vi "Initialize.vi"(8 "error in":errorcluster, 10 "Btr0Btr1":u16=28 format="%.0x", 11 "Channel":u16=65 format="%x") -> (0 "error out":errorcluster, 3 "Channel out":u16=81, 5 "function return":u32)   [LabVIEW 2023, in "PCAN API.lvlib"]
doc: "This VI is used for initializing a CAN port."
uses:
  PCAN API.lvlib
  PCAN2023/PCAN2023.lvlib
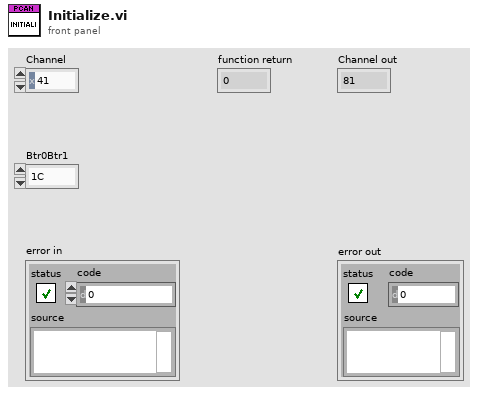
[diagram p1: front panel]
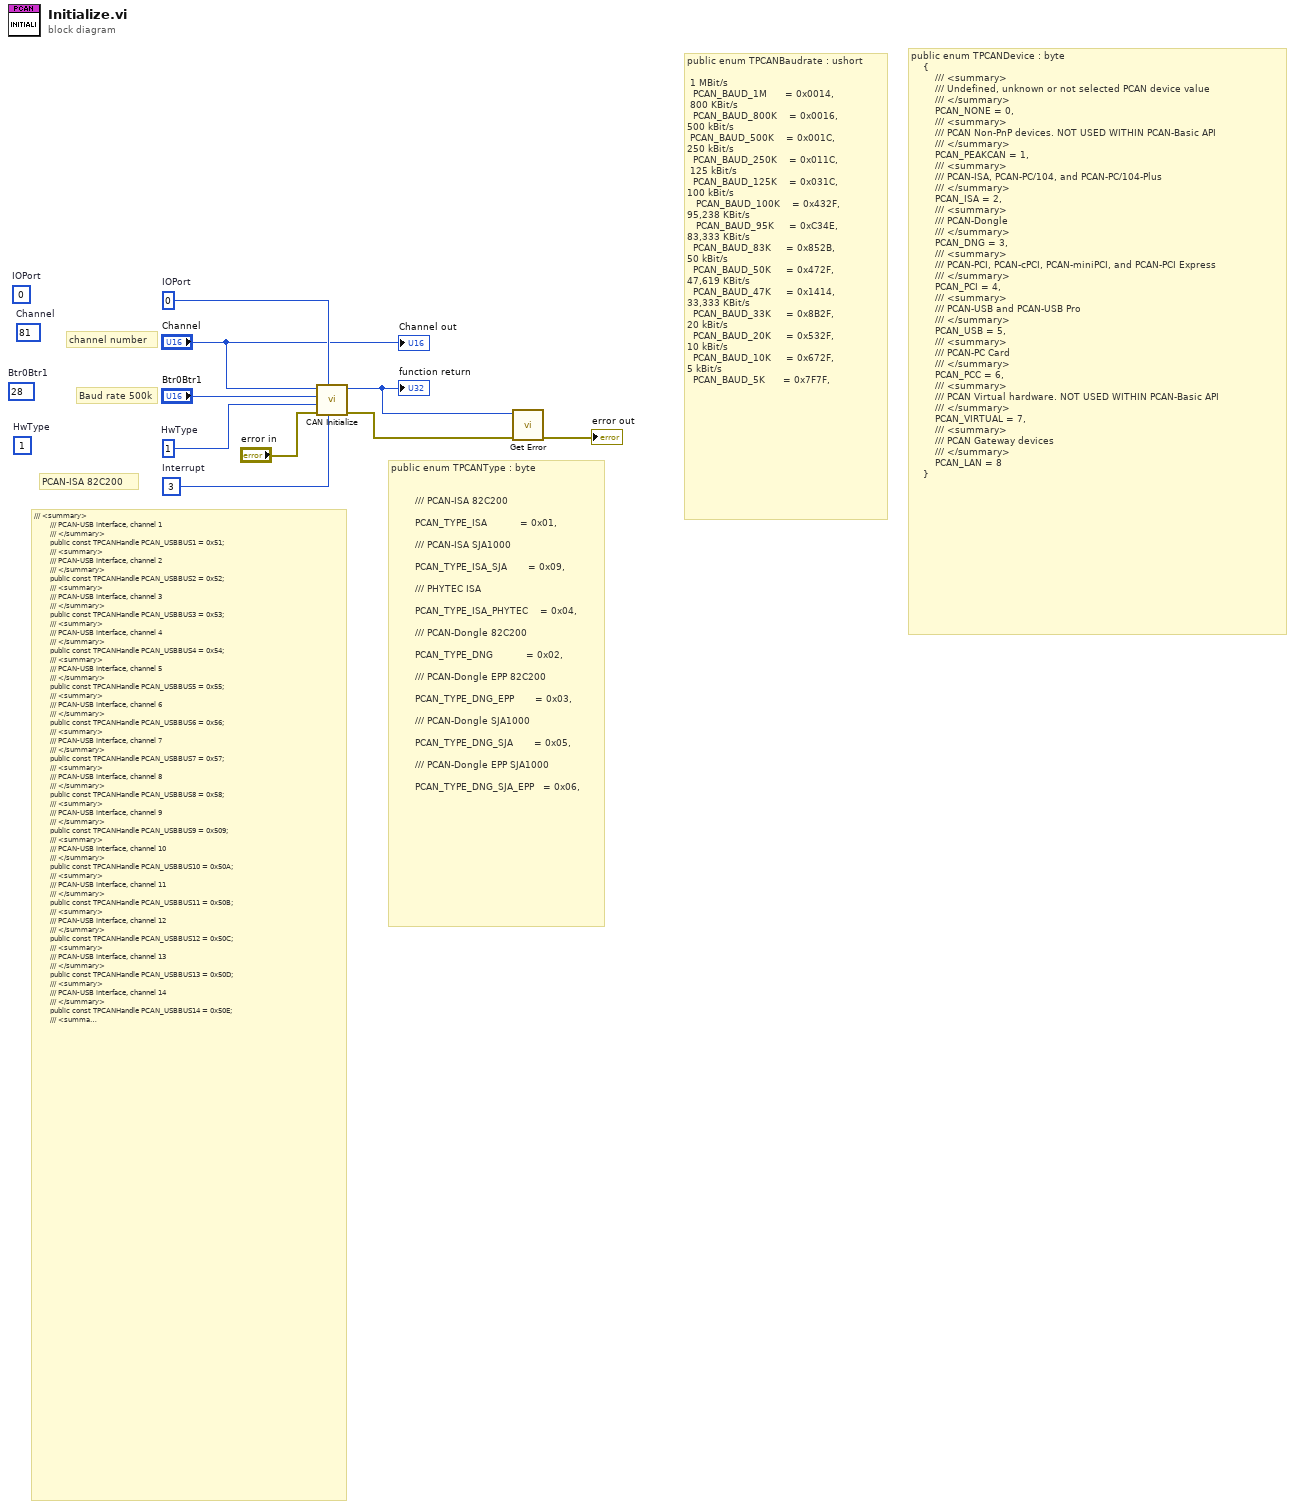
[diagram p0: block diagram]
diagram:
  w6 = u8 1  # HwType
  w9 = u32 0  # IOPort
  (unwired) u16 28  # Btr0Btr1
  (unwired) u8 1  # HwType
  (unwired) u32 0  # IOPort
  (unwired) u16 81  # Channel
  w8 = u16 3  # Interrupt
  # "/// <summary>\n        /// PCAN-USB interface, channel 1\n        /// </summary>\n        public const TPCANHandle PCAN_USBBUS1 = 0x51;\n        /// <summary>\n        /// PCAN-USB interface, channel 2\n        /// </summary>\n        public const TPCANHandle PCAN_USBBUS2 = 0x52;\n        /// <summary>\n        /// PCAN-USB interface, channel 3\n        /// </summary>\n        public const TPCANHandle PCAN_USBBUS3 = 0x53;\n        /// <summary>\n        /// PCAN-USB interface, channel 4\n        /// </summary>\n        public const TPCANHandle PCAN_USBBUS4 = 0x54;\n        /// <summary>\n        /// PCAN-USB interface, channel 5\n        /// </summary>\n        public const TPCANHandle PCAN_USBBUS5 = 0x55;\n        /// <summary>\n        /// PCAN-USB interface, channel 6\n        /// </summary>\n        public const TPCANHandle PCAN_USBBUS6 = 0x56;\n        /// <summary>\n        /// PCAN-USB interface, channel 7\n        /// </summary>\n        public const TPCANHandle PCAN_USBBUS7 = 0x57;\n        /// <summary>\n        /// PCAN-USB interface, channel 8\n        /// </summary>\n        public const TPCANHandle PCAN_USBBUS8 = 0x58;\n        /// <summary>\n        /// PCAN-USB interface, channel 9\n        /// </summary>\n        public const TPCANHandle PCAN_USBBUS9 = 0x509;\n        /// <summary>\n        /// PCAN-USB interface, channel 10\n        /// </summary>\n        public const TPCANHandle PCAN_USBBUS10 = 0x50A;\n        /// <summary>\n        /// PCAN-USB interface, channel 11\n        /// </summary>\n        public const TPCANHandle PCAN_USBBUS11 = 0x50B;\n        /// <summary>\n        /// PCAN-USB interface, channel 12\n        /// </summary>\n        public const TPCANHandle PCAN_USBBUS12 = 0x50C;\n        /// <summary>\n        /// PCAN-USB interface, channel 13\n        /// </summary>\n        public const TPCANHandle PCAN_USBBUS13 = 0x50D;\n        /// <summary>\n        /// PCAN-USB interface, channel 14\n        /// </summary>\n        public const TPCANHandle PCAN_USBBUS14 = 0x50E;\n        /// <summary>\n        /// PCAN-USB interface, channel 15\n        /// </summary>\n        public const TPCANHandle PCAN_USBBUS15 = 0x50F;\n        /// <summary>\n        /// PCAN-USB interface, channel 16\n        /// </summary>\n        public const TPCANHandle PCAN_USBBUS16 = 0x510;\n\n        /// <summary>"
  # "public enum TPCANType : byte\n\n\n        /// PCAN-ISA 82C200\n\n        PCAN_TYPE_ISA           = 0x01,\n\n        /// PCAN-ISA SJA1000\n\n        PCAN_TYPE_ISA_SJA       = 0x09,\n\n        /// PHYTEC ISA \n\n        PCAN_TYPE_ISA_PHYTEC    = 0x04,\n\n        /// PCAN-Dongle 82C200\n \n        PCAN_TYPE_DNG           = 0x02,\n\n        /// PCAN-Dongle EPP 82C200\n\n        PCAN_TYPE_DNG_EPP       = 0x03,\n\n        /// PCAN-Dongle SJA1000\n\n        PCAN_TYPE_DNG_SJA       = 0x05,\n    \n        /// PCAN-Dongle EPP SJA1000\n\n        PCAN_TYPE_DNG_SJA_EPP   = 0x06,"
  # "public enum TPCANDevice : byte\n    {\n        /// <summary>\n        /// Undefined, unknown or not selected PCAN device value\n        /// </summary>\n        PCAN_NONE = 0,\n        /// <summary>\n        /// PCAN Non-PnP devices. NOT USED WITHIN PCAN-Basic API\n        /// </summary>\n        PCAN_PEAKCAN = 1,\n        /// <summary>\n        /// PCAN-ISA, PCAN-PC/104, and PCAN-PC/104-Plus\n        /// </summary>\n        PCAN_ISA = 2,\n        /// <summary>\n        /// PCAN-Dongle\n        /// </summary>\n        PCAN_DNG = 3,\n        /// <summary>\n        /// PCAN-PCI, PCAN-cPCI, PCAN-miniPCI, and PCAN-PCI Express\n        /// </summary>\n        PCAN_PCI = 4,\n        /// <summary>\n        /// PCAN-USB and PCAN-USB Pro\n        /// </summary>\n        PCAN_USB = 5,\n        /// <summary>\n        /// PCAN-PC Card\n        /// </summary>\n        PCAN_PCC = 6,\n        /// <summary>\n        /// PCAN Virtual hardware. NOT USED WITHIN PCAN-Basic API\n        /// </summary>\n        PCAN_VIRTUAL = 7,\n        /// <summary>\n        /// PCAN Gateway devices\n        /// </summary>\n        PCAN_LAN = 8\n    }"
  # "public enum TPCANBaudrate : ushort\n\n 1 MBit/s\n  PCAN_BAUD_1M      = 0x0014,\n 800 KBit/s\n  PCAN_BAUD_800K    = 0x0016,\n500 kBit/s\n PCAN_BAUD_500K    = 0x001C,\n250 kBit/s\n  PCAN_BAUD_250K    = 0x011C,\n 125 kBit/s\n  PCAN_BAUD_125K    = 0x031C,\n100 kBit/s\n   PCAN_BAUD_100K    = 0x432F,\n95,238 KBit/s\n   PCAN_BAUD_95K     = 0xC34E,\n83,333 KBit/s\n  PCAN_BAUD_83K     = 0x852B,\n50 kBit/s\n  PCAN_BAUD_50K     = 0x472F,\n47,619 KBit/s\n  PCAN_BAUD_47K     = 0x1414,\n33,333 KBit/s\n  PCAN_BAUD_33K     = 0x8B2F,\n20 kBit/s\n  PCAN_BAUD_20K     = 0x532F,\n10 kBit/s\n  PCAN_BAUD_10K     = 0x672F,\n5 kBit/s\n  PCAN_BAUD_5K      = 0x7F7F,"
  # "channel number"
  # "PCAN-ISA 82C200"
  # "Baud rate 500k"
  n1 = call "CAN Initialize.vi"("Interrupt"=w8, "IOPort"=w9, "error in (no error)"="error in", "HwType"=w6, "Btr0Btr1"="Btr0Btr1", "Channel"="Channel") -> ("error out"=w1:errorcluster, "function return"=w3:u32)  [unwired: 4 in]
  "function return" <- w3
  n2 = call "Get Error.vi"("error in (no error)"=w1, "function return"=w3) -> ("error out"=→"error out":errorcluster)  [unwired: 9 in]
  "Channel out" <- "Channel"
